vi "Filter Errors.vi"(0 "Filtered Errors":i32[](array[numeric]), 3 "error in (no error)":errorcluster) -> (9 "error out":errorcluster)   [LabVIEW 2021, in "Error.lvlib"]
uses:
  <vilib>/ErrorRing/Error Ring.xnode
  Error.lvlib
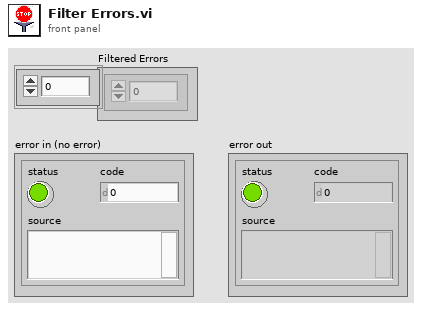
[diagram p1: front panel]
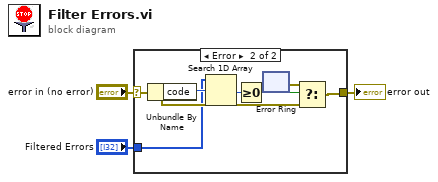
[diagram p0: block diagram]
diagram:
  n1 = case shown="Error" "error in (no error)" {
    selector: "error in (no error)" -> [w4 w9]
    tunnel: [w4 w11] -> w2
    tunnel: "Filtered Errors" -> [_ w5]
    frame No Error {
    }
    frame Error {
      n2 = Unbundle By Name(w9) -> ("code"=w8:i32)
      n3 = Search 1D Array(1D array=w5, element=w8) -> (index of element=w7:i32)  [unwired: 1 in]
      n4 = Greater Or Equal To 0?(x=w7) -> (x >= 0?=w6:bool)
      n5 = xnode "Error Ring"() -> ("error out"=w10:errorcluster)
      n6 = Select(t=w10, s=w6, f=w9) -> (s? t:f=w11:errorcluster)
    }
  }
  "error out" <- w2
